vi "FGV_MG_Frequency.vi"(6 "Buffer Size":i32=10000, 7 "Command":T1, 8 "error in (no error)":errorcluster, 11 "Sample":fxp<+,32,8>) -> (0 "error out":errorcluster, 3 "Buffer":fxp<+,32,8>[](array[numeric]), 5 "Buffer Index":i32)   [LabVIEW 2015]
uses:
  Data_Queue_Command.ctl
panel:
  # "32,8"
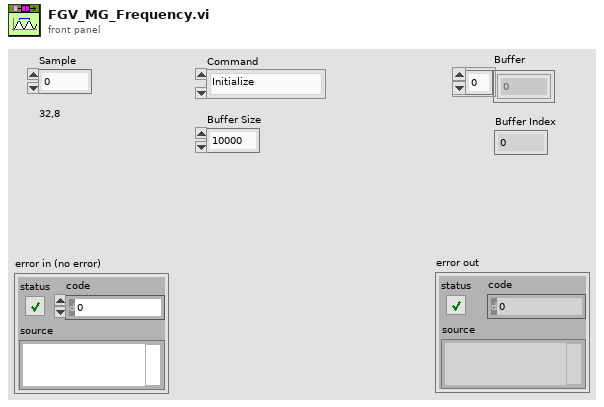
[diagram p1: front panel]
types:
  T1 = typedef "Data_Queue_Command.ctl" = enum16{"Initialize", "Write Sample", "Pull Array", "Close"}
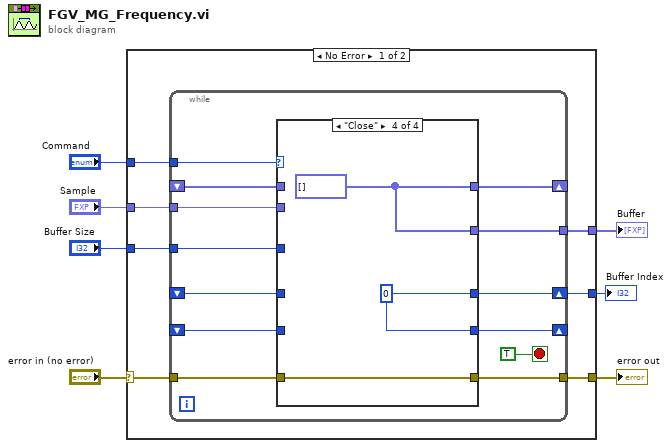
[diagram p0: block diagram]
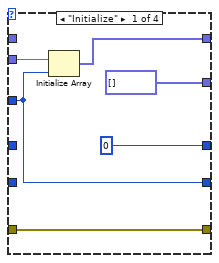
[diagram p2: hidden frame]
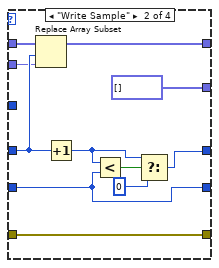
[diagram p3: hidden frame]
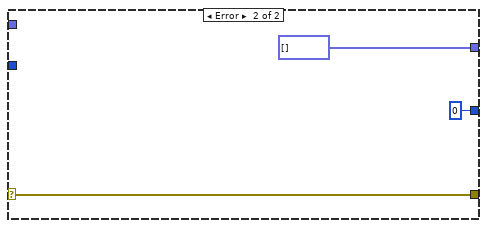
[diagram p5: hidden frame]
diagram:
  n1 = case shown="No Error" "error in (no error)" {
    selector: "error in (no error)" -> [w10 w54]
    tunnel: [w9 w54] -> w6
    tunnel: "Command" -> [w14 _]
    tunnel: "Buffer Size" -> [w13 _]
    tunnel: "Sample" -> [w12 _]
    tunnel: [w11 fxp<+,32,8>[] []] -> w2
    tunnel: [w8 0 ("f")] -> w1
    frame No Error {
      n2 = while {
        tunnel: w14 -> [w26]
        tunnel: w13 -> [w25]
        tunnel: w12 -> [w24]
        shift-right: [w23] -> _
        shift-left: _ -> [w22]
        shift-right: [w21] -> _
        shift-left: _ -> [w20]
        shift-right: [w19] -> w8
        shift-left: _ -> [w18]
        tunnel: [w17] -> w11
        tunnel: w10 -> [w16]
        tunnel: [w15] -> w9
        stop <- TRUE stop-if-true
        n3 = case shown="\"Close\"" w26 {
          tunnel: w25 -> [w31 _ _ _]
          tunnel: w24 -> [w33 w37 _ _]
          tunnel: [w32 w38 w46 w51] -> w23
          tunnel: w22 -> [_ w44 w46 _]
          tunnel: [w31 w36 w47 w50] -> w21
          tunnel: w20 -> [_ w36 w47 _]
          tunnel: [0 ("Buffer Index") w39 w48 w50] -> w19
          tunnel: w18 -> [_ w43 w48 _]
          tunnel: [fxp<+,32,8>[] [] fxp<+,32,8>[] [] w46 w51] -> w17
          tunnel: w16 -> [w28 w34 w45 w49]
          tunnel: [w28 w34 w45 w49] -> w15
          frame "Initialize" {
            n4 = Initialize Array(w33, w31) -> (w32:fxp<+,32,8>[])
          }
          frame "Write Sample" {
            n5 = Replace Array Subset(array=w44, new element=w37, index=w43) -> (w38:fxp<+,32,8>[])
            n6 = Increment(x=w43) -> (x+1=w41:i32)
            n7 = Less?(x=w41, y=w36) -> (x < y?=w42:bool)
            n8 = Select(t=w41, s=w42, f=0) -> (s? t:f=w39:i32)
          }
          frame "Pull Array" {
          }
          frame "Close" {
            w50 = 0 ("f")
            w51 = fxp<+,32,8>[] []
          }
        }
      }
    }
    frame Error {
    }
  }
  "Buffer" <- w2
  "error out" <- w6
  "Buffer Index" <- w1
